vi "WFM data to file packet.vi"(6 "Save RPM Data":bool, 11 "WFM Data In":waveform(dbl)[](array[waveform])) -> (2 "Header":string, 3 "Data Out":string[][](array[string]))   [LabVIEW 2017]
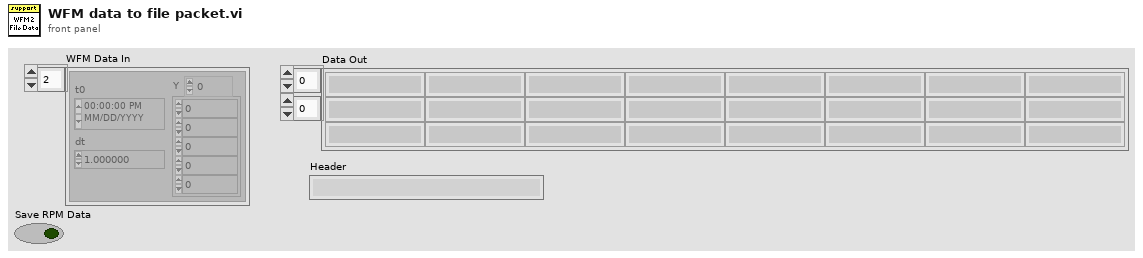
[diagram p1: front panel]
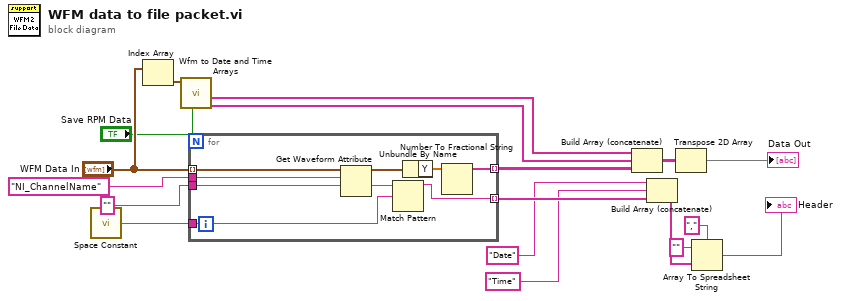
[diagram p0: block diagram]
diagram:
  n1 = call <vilib>:"Space Constant.vi"() -> ("String"=w10:string)
  n2 = Index Array(array="WFM Data In") -> (element=w18:waveform(dbl))  [unwired: 1 in]
  n3 = call "Wfm to Date and Time Arrays.vi"("Save RPM Data"="Save RPM Data", "Wfm In"=w18) -> ("Time Strings"=w14:string[], "Date Strings"=w15:string[])  [unwired: 8 in]
  n4 = for {
    tunnel: "WFM Data In" -> [w25] mode=indexing
    tunnel: [w26] -> w16 mode=indexing
    tunnel: "NI_ChannelName" ("name") -> [w23]
    tunnel: "" -> [w22]
    tunnel: [w20] -> w9 mode=indexing
    tunnel: w10 -> [w19]
    n5 = Get Waveform Attribute(5:w22, 6:w23, 7:w25) -> (1:w21:string, 3:w24:waveform(dbl))  [unwired: 1 in, 2 out]
    n6 = Match Pattern(string=w21, regular expression=w19) -> (before substring=w20:string)  [unwired: 1 in, 3 out]
    n7 = Unbundle By Name(w24) -> ("Y"=w27:dbl[])
    n8 = Number To Fractional String(number=w27) -> (F-format string=w26:string[])  [unwired: 3 in]
  }
  n9 = Build Array (concatenate)(w15, w14, w16) -> (w13:string[][])
  n10 = Build Array (concatenate)("Date", "Time", w9) -> (w5:string[])
  n11 = Transpose 2D Array(2D array=w13) -> (transposed array=→"Data Out":string[][])
  n12 = Array To Spreadsheet String(delimiter (Tab)=",", array=w5, 3:"" ("format string")) -> (spreadsheet string=→"Header":string)
